vi "SortEnableButtons.vi"(10 "Radio Buttons":T1=enum."Step 1") -> (1 "Enable out":T2, 2 "FilterStage":u8, 3 "EnableStep1 out":bool)   [LabVIEW 2018]
uses:
  Controls/Clusts/FPGA_Filter_Enable.ctl
  Controls/RadioButtons/FilterEnableRadio.ctl
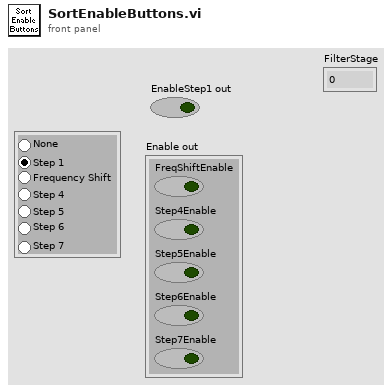
[diagram p1: front panel]
types:
  T1 = typedef "FilterEnableRadio.ctl" = enum32{"None", "Step 1", "Frequency Shift", "Step 4", "Step 5", "Step 6", "Step 7"}
  T2 = typedef "FPGA_Filter_Enable.ctl" = cluster{"FreqShiftEnable":bool, "Step4Enable":bool, "Step5Enable":bool, "Step6Enable":bool, "Step7Enable":bool}
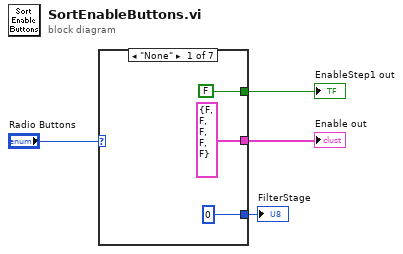
[diagram p0: block diagram]
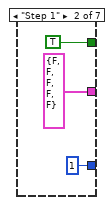
[diagram p2: hidden frame]
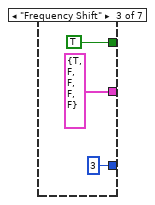
[diagram p3: hidden frame]
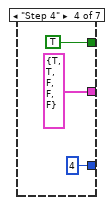
[diagram p4: hidden frame]
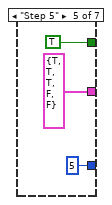
[diagram p5: hidden frame]
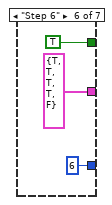
[diagram p6: hidden frame]
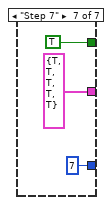
[diagram p7: hidden frame]
diagram:
  n1 = case shown="\"None\"" "Radio Buttons" {
    tunnel: [T2 {"FreqShiftEnable"=FALSE, "Step4Enable"=FALSE, "Step5Enable"=FALSE, "Step6Enable"=FALSE, "Step7Enable"=FALSE} ("Enable in") T2 {"FreqShiftEnable"=FALSE, "Step4Enable"=FALSE, "Step5Enable"=FALSE, "Step6Enable"=FALSE, "Step7Enable"=FALSE} ("Enable in") T2 {"FreqShiftEnable"=TRUE, "Step4Enable"=FALSE, "Step5Enable"=FALSE, "Step6Enable"=FALSE, "Step7Enable"=FALSE} ("Enable in") T2 {"FreqShiftEnable"=TRUE, "Step4Enable"=TRUE, "Step5Enable"=FALSE, "Step6Enable"=FALSE, "Step7Enable"=FALSE} ("Enable in") T2 {"FreqShiftEnable"=TRUE, "Step4Enable"=TRUE, "Step5Enable"=TRUE, "Step6Enable"=FALSE, "Step7Enable"=FALSE} ("Enable in") T2 {"FreqShiftEnable"=TRUE, "Step4Enable"=TRUE, "Step5Enable"=TRUE, "Step6Enable"=TRUE, "Step7Enable"=FALSE} ("Enable in") T2 {"FreqShiftEnable"=TRUE, "Step4Enable"=TRUE, "Step5Enable"=TRUE, "Step6Enable"=TRUE, "Step7Enable"=TRUE} ("Enable in")] -> w4
    tunnel: [FALSE ("EnableStep1 in") TRUE ("EnableStep1 in") TRUE ("EnableStep1 in") TRUE ("EnableStep1 in") TRUE ("EnableStep1 in") TRUE ("EnableStep1 in") TRUE ("EnableStep1 in")] -> w3
    tunnel: [u8 0 u8 1 u8 3 u8 4 u8 5 u8 6 u8 7] -> w1
    frame "None" {
    }
    frame "Step 1" {
    }
    frame "Frequency Shift" {
    }
    frame "Step 4" {
    }
    frame "Step 5" {
    }
    frame "Step 6" {
    }
    frame "Step 7" {
    }
  }
  "Enable out" <- w4
  "EnableStep1 out" <- w3
  "FilterStage" <- w1
